vi "WPI_Camera HTTP Connection Respondervi.vi"(10 "parameters":T1(array[cluster]), 11 "connection ID":refnum<k5>) -> ()   [LabVIEW 2017]
doc: "This VI is launched each time a new client camera connection is requested. The connection will remain open until closed by the client or because of errors with the camera. Parameters are name/lvalue pairs that have been parsed from a URL request. Supported parameters are name, fps, resolution, compression, exposure, brightness, whitebalance, sharpness, and colorlevel.\n\nThe first four parameters are filled with defaults if not provided, but the latter four are only set if provided."
uses:
  <vilib>/Rock Robotics/SystemInterfaces/NetworkCommunication/NetComm_UsageReport_ResourceType.ctl
  <vilib>/Rock Robotics/WPI/Camera/WPI_CameraImageSize.ctl
  <vilib>/Utility/error.llb/Error Cluster From Error Code.vi
  <vilib>/ErrorRing/Error Ring.xnode
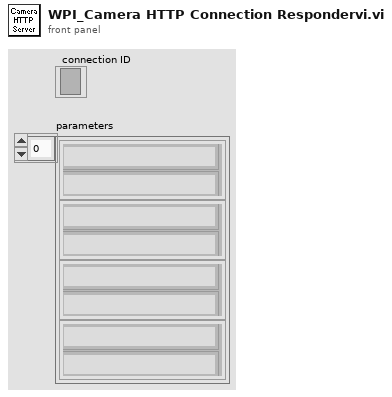
[diagram p1: front panel]
types:
  T1 = cluster{"token string":string, "token string 2":string}[]
  T2 = typedef "Image Type" = u32
  T3 = cluster{"White Balance":string, "Brightness":i32, "Sharpness":i32, "Saturation":i32, "Exposure":string}
  T4 = cluster{"Camera Name":string, "Size":string, "Frame Rate":i32, "Compression":i32}
  T5 = typedef "NetComm_UsageReport_ResourceType.ctl" = enum8{"Controller", "Module", "Language", "CANPlugin", "Accelerometer", "ADXL345", "AnalogChannel", "AnalogTrigger", "AnalogTriggerOutput", "CANJaguar", "Compressor", "Counter", "Dashboard", "DigitalInput", "DigitalOutput", "DriverStationCIO", "DriverStationEIO", "DriverStationLCD", "Encoder", "GearTooth", "Gyro", "I2C", "Framework", "Jaguar", "Joystick", "Kinect", "KinectStick", "PIDController", "Preferences", "PWM", "Relay", "RobotDrive", "SerialPort", "Servo", "Solenoid", "SPI", "Task", "Ultrasonic", "Victor", "Button", "Command", "AxisCamera", "PCVideoServer", "SmartDashboard", "Talon", "HiTechnicColorSensor", "HiTechnicAccel", "HiTechnicCompass", "SRF08", "AnalogOutput", "Victor SP", "Talon SRX", "CAN Talon SRX", "ADXL362 Accel", "ADXRS450 Gyro", "Rev SPARK", "Mindsensors SD540", "Digital Filter", "ADIS16448", "PDP", "PCM", "PigeonIMU", "Nidec Brushless", "CTRE CANifier", "CTRE Future 0", "CTRE Future 1", "CTRE Future 2", "CTRE Future 3", "CTRE Future 4", "CTRE Future 5", "CTRE Future 6"}
  T6 = cluster{"White Balance":bool, "Brightness":bool, "Sharpness":bool, "Saturation":bool, "Exposure":bool}
  T7 = typedef "WPI_CameraDevRef.ctl" = cluster{"Camera Address":string, "CameraStatus":errorcluster}
  T8 = typedef "IMAQ Image.ctl" = refnum<image>
  T9 = typedef "WPI_CameraImageSize.ctl" = enum16{"640x480", "320x240", "160x120", "Custom"}
  T10 = enum16{"Update Mode", "Get Image", "Get Image Data"}
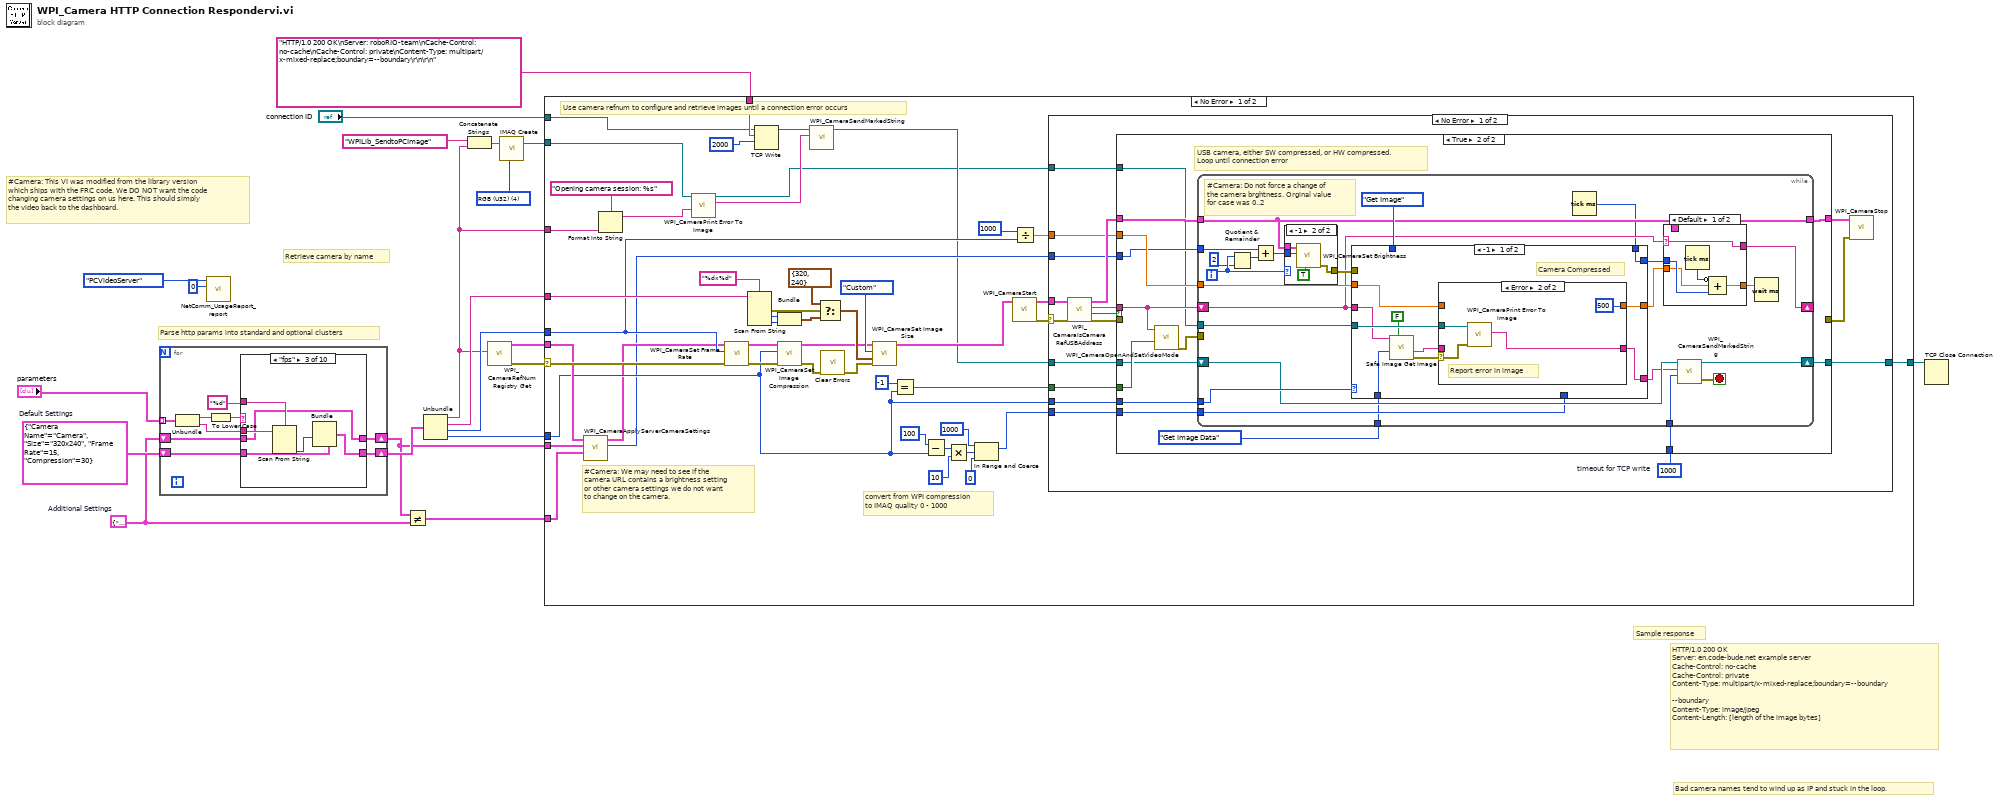
[diagram p0: block diagram]
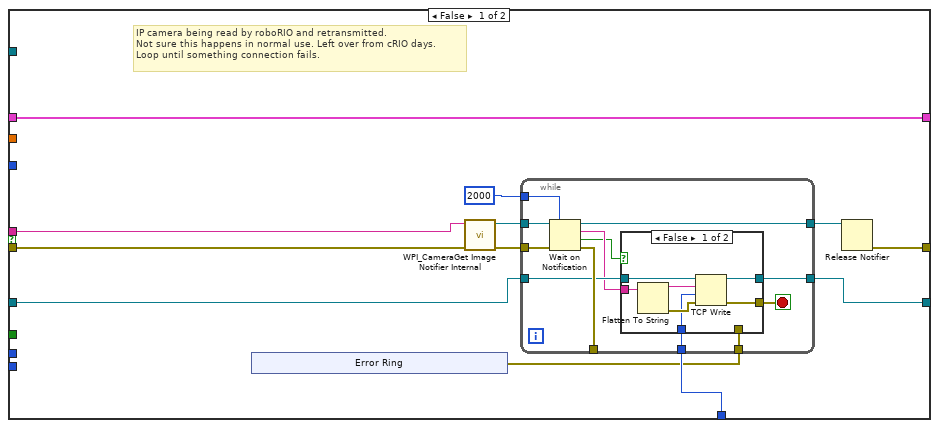
[diagram p2: hidden frame]
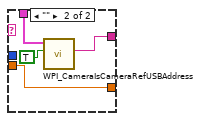
[diagram p4: hidden frame]
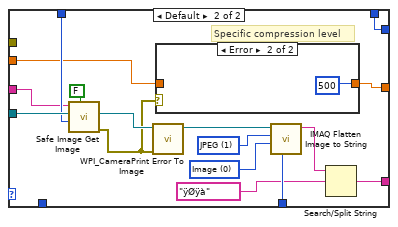
[diagram p7: hidden frame]
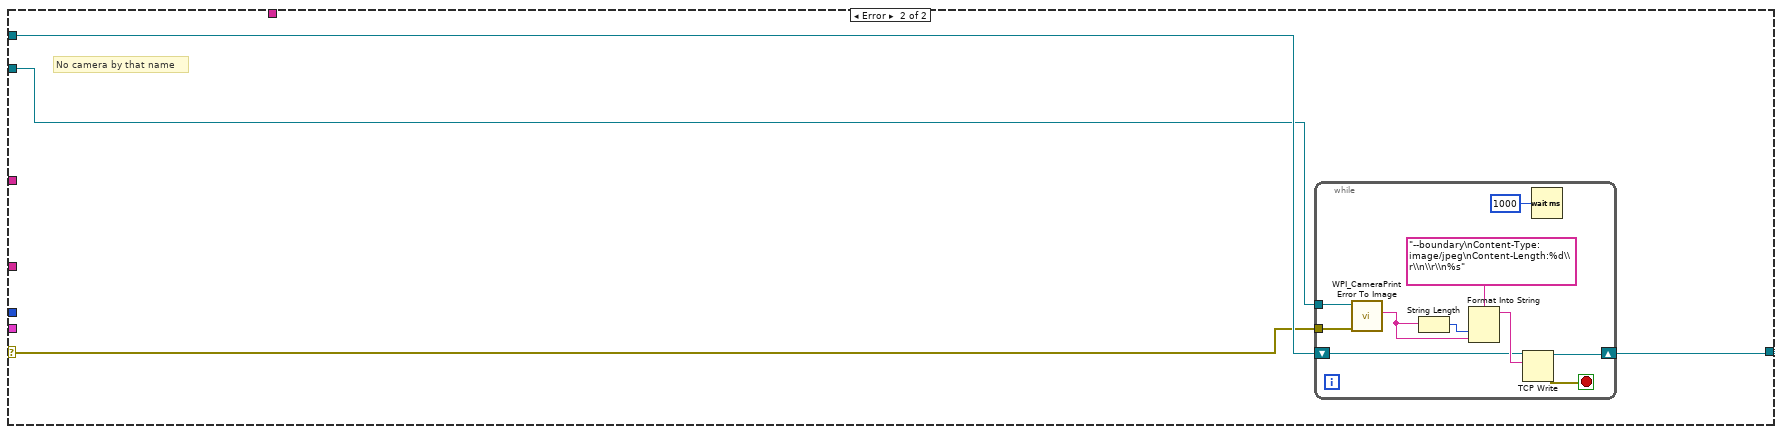
[diagram p10: hidden frame]
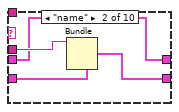
[diagram p12: hidden frame]
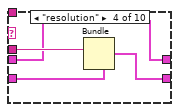
[diagram p13: hidden frame]
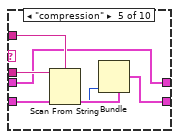
[diagram p14: hidden frame]
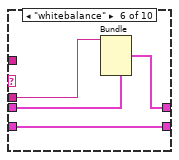
[diagram p15: hidden frame]
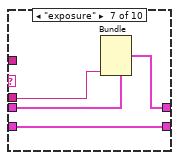
[diagram p16: hidden frame]
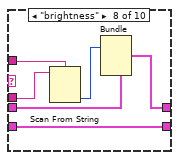
[diagram p17: hidden frame]
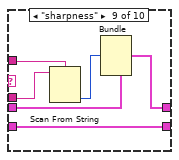
[diagram p18: hidden frame]
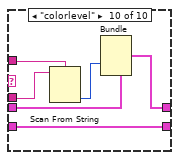
[diagram p19: hidden frame]
diagram:
  w4 = T2 4 items=["Grayscale (U8)", "Grayscale (I16)", "Grayscale (SGL)", "Complex (CSG)", "RGB (U32)", "HSL (U32)", "RGB (U64)", "Grayscale (U16)"] ("Image Type")
  w12 = T3 {"White Balance"="", "Brightness"=-1, "Sharpness"=-1, "Saturation"=-1, "Exposure"=""}  # Additional Settings
  w18 = T4 {"Camera Name"="Camera", "Size"="320x240", "Frame Rate"=15, "Compression"=30}  # Default Settings
  # "#Camera: This VI was modified from the library version\nwhich ships with the FRC code. We DO NOT want the code\nchanging camera settings on us here. This should simply\nthe video back to the dashboard."
  # "Sample response"
  # "HTTP/1.0 200 OK\nServer: en.code-bude.net example server\nCache-Control: no-cache\nCache-Control: private\nContent-Type: multipart/x-mixed-replace;boundary=--boundary\n \n--boundary\nContent-Type: image/jpeg\nContent-Length: [length of the image bytes]"
  # "Retrieve camera by name"
  # "Parse http params into standard and optional clusters"
  # "Bad camera names tend to wind up as IP and stuck in the loop."
  n1 = for {
    tunnel: "parameters" -> [w30] mode=indexing
    shift-right: [w25] -> w15
    shift-left: w18 -> [w27]
    shift-right: [w22] -> w10
    shift-left: w12 -> [w23]
    n2 = Unbundle(w30) -> ("token string"=w29:string, "token string 2"=w26:string)
    n3 = To Lower Case(string=w29) -> (all lower case string=w28:string)
    n4 = case shown="\"fps\"" w28 {
      tunnel: w27 -> [w32 w36 w42 w46 w52 w56 w60 w66 w72 w78]
      tunnel: w26 -> [_ w35 w40 w44 w50 w54 w57 w62 w68 w74]
      tunnel: [w32 w34 w41 w45 w51 w56 w60 w66 w72 w78] -> w25
      tunnel: "%d" -> [_ _ w39 _ w48 _ _ w63 w69 w75]
      tunnel: w23 -> [w31 w33 w37 w43 w47 w55 w59 w65 w71 w77]
      tunnel: [w31 w33 w37 w43 w47 w53 w58 w64 w70 w76] -> w22
      frame Default {
      }
      frame "name" {
        n5 = Bundle(cluster=w36, "Camera Name"=w35) -> (w34:T4)  [unwired: 3 in]
      }
      frame "fps" {
        n6 = Scan From String(format string=w39, input string=w40) -> (output 1=w38:i32)  [unwired: 3 in, 3 out]
        n7 = Bundle(cluster=w42, "Frame Rate"=w38) -> (w41:T4)  [unwired: 3 in]
      }
      frame "resolution" {
        n8 = Bundle(cluster=w46, "Size"=w44) -> (w45:T4)  [unwired: 3 in]
      }
      frame "compression" {
        n9 = Scan From String(format string=w48, input string=w50) -> (output 1=w49:i32)  [unwired: 3 in, 3 out]
        n10 = Bundle(cluster=w52, "Compression"=w49) -> (w51:T4)  [unwired: 3 in]
      }
      frame "whitebalance" {
        n11 = Bundle(cluster=w55, "White Balance"=w54) -> (w53:T3)  [unwired: 4 in]
      }
      frame "exposure" {
        n12 = Bundle(cluster=w59, "Exposure"=w57) -> (w58:T3)  [unwired: 4 in]
      }
      frame "brightness" {
        n13 = Scan From String(format string=w63, input string=w62) -> (output 1=w61:i32)  [unwired: 3 in, 3 out]
        n14 = Bundle(cluster=w65, "Brightness"=w61) -> (w64:T3)  [unwired: 4 in]
      }
      frame "sharpness" {
        n15 = Scan From String(format string=w69, input string=w68) -> (output 1=w67:i32)  [unwired: 3 in, 3 out]
        n16 = Bundle(cluster=w71, "Sharpness"=w67) -> (w70:T3)  [unwired: 4 in]
      }
      frame "colorlevel" {
        n17 = Scan From String(format string=w75, input string=w74) -> (output 1=w73:i32)  [unwired: 3 in, 3 out]
        n18 = Bundle(cluster=w77, "Saturation"=w73) -> (w76:T3)  [unwired: 4 in]
      }
    }
  }
  n19 = call <vilib>:"NetComm_UsageReport_report.vi"("Instance Number"=u8 0, "Resource Type"=NetComm_UsageReport_ResourceType."PCVideoServer") -> ()  [unwired: 10 in]
  n20 = Not Equal?(x=w10, y=w12) -> (x != y?=w11:T6)
  n21 = Unbundle(w15) -> ("Camera Name"=w2:string, "Size"=w16:string, "Frame Rate"=w8:i32, "Compression"=w9:i32)
  n22 = Concatenate Strings("WPILib_SendtoPCImage", w2) -> (w3:string)
  n23 = call <vilib>:"WPI_CameraRefNum Registry Get.vi"("refnum name"=w2) -> ("error out"=w6:errorcluster, "CameraDevRef"=w17:T7)  [unwired: 9 in]
  n24 = call "IMAQ Create"("Image Name"=w3, "Image Type"=w4) -> ("New Image"=w5:T8)  [unwired: 3 in, 1 out]
  n25 = case shown="No Error" w6 {
    selector: w6 -> [w102 w268]
    tunnel: [w126 w269] -> w21
    tunnel: w17 -> [w94 _]
    tunnel: w16 -> [w113 _]
    tunnel: w11 -> [w104 _]
    tunnel: w10 -> [w103 _]
    tunnel: w9 -> [w93 _]
    tunnel: w8 -> [w101 _]
    tunnel: "connection ID" -> [w81 w270]
    tunnel: w5 -> [w86 w267]
    tunnel: w2 -> [w88 _]
    tunnel: "HTTP/1.0 200 OK\nServer: roboRIO-team\nCache-Control: no-cache\nCache-Control: private\nContent-Type: multipart/x-mixed-replace;boundary=--boundary\r\n\r\n" ("regular expression") -> [w82 _]
    frame No Error {
      # "#Camera: We may need to see if the\ncamera URL contains a brightness setting\nor other camera settings we do not want\nto change on the camera."
      # "Use camera refnum to configure and retrieve images until a connection error occurs"
      # "convert from WPI compression\nto IMAQ quality 0 - 1000"
      n26 = call <vilib>:"WPI_CameraApplyServerCameraSettings.vi"("Unique"=w104, "Additional Settings"=w103, "CameraDevRef"=w94) -> ("Brightness"=w91:i32, "CameraDevRef Out"=w92:T7)  [unwired: 7 in]
      n27 = Format Into String(format string="Opening camera session: %s", w88) -> (resulting string=w84:string)  [unwired: 2 in, 1 out]
      n28 = call <vilib>:"WPI_CameraPrint Error To Image.vi"("String"=w84, "Image"=w86) -> ("flattened error string"=w90:string, "Image out"=w85:T8)  [unwired: 8 in]
      n29 = call <vilib>:"WPI_CameraSet Frame Rate.vi"("error in (no error)"=w102, "Frame Rate (fps)"=w101, "CameraDevRef"=w92) -> ("error out"=w98:errorcluster, "CameraDevRef Out"=w100:T7)  [unwired: 7 in]
      n30 = Scan From String(format string="%dx%d", input string=w113) -> (error out=w108:errorcluster, output 1=w111:i32, output 2=w110:i32)  [unwired: 4 in, 2 out]
      n31 = TCP Write(connection ID=w81, data in=w82, 9:2000) -> (connection ID out=w80:refnum<k5>)  [unwired: 1 in, 2 out]
      n32 = Bundle(w111, w110) -> (w107:cluster{i32, i32})  [unwired: 1 in]
      n33 = call <vilib>:"WPI_CameraSet Image Compression.vi"("error in (no error)"=w98, "Compression"=w93, "CameraDevRef"=w100) -> ("error out"=w97:errorcluster, "CameraDevRef Out"=w99:T7)  [unwired: 7 in]
      n34 = call <vilib>:"WPI_CameraSendMarkedString.vi"("Data String"=w90, "TCP Network Connection in"=w80) -> ("TCP Network Connection out"=w89:refnum<k5>)  [unwired: 8 in, 1 out]
      n35 = Select(t=cluster{i32, i32} {320, 240} ("s? t:f"), s=w108, f=w107) -> (s? t:f=w106:cluster{i32, i32})
      n36 = call <vilib>:"Clear Errors.vi"("error in (no error)"=w97) -> ("error out"=w96:errorcluster)  [unwired: 5 in, 1 out]
      n37 = call <vilib>:"WPI_CameraSet Image Size.vi"("error in (no error)"=w96, "Size W,H (pix)"=w106, "Image Size"=WPI_CameraImageSize."Custom", "CameraDevRef"=w99) -> ("CameraDevRef Out"=w95:T7)  [unwired: 6 in, 1 out]
      n38 = Equal?(x=-1, y=w93) -> (x = y?=w114:bool)
      n39 = Subtract(x=100, y=w93) -> (x-y=w118:i32)
      n40 = Multiply(x=w118, y=10) -> (x*y=w120:i32)
      n41 = In Range and Coerce(upper limit=1000, x=w120, lower limit=0) -> (coerced(x)=w116:i32)  [unwired: 1 out]
      n42 = call <vilib>:"WPI_CameraStart.vi"("CameraDevRef"=w95) -> ("error out"=w79:errorcluster, "CameraDevRef"=w125:T7)  [unwired: 1 in, 8 out]
      n43 = Divide(x=u16 1000 ("port"), y=w101) -> (x/y=w123:dbl)
      n44 = case shown="No Error" w79 {
        selector: w79 -> [w127 _]
        tunnel: [w143 w266] -> w126
        tunnel: w125 -> [w138 _]
        tunnel: w123 -> [w136 _]
        tunnel: w116 -> [w135 _]
        tunnel: w114 -> [w134 _]
        tunnel: w93 -> [w131 _]
        tunnel: w91 -> [w130 _]
        tunnel: w89 -> [w129 w266]
        tunnel: w85 -> [w128 _]
        frame No Error {
          w132 = 1000  # timeout for TCP write
          n45 = call <vilib>:"WPI_CameraIsCameraRefUSBAddress.vi"("error in (no error)"=w127, "CameraDevRef"=w138) -> ("error out"=w133:errorcluster, "USB?"=w139:bool, "Camera Address Out"=w140:string, "CameraDevRef out"=w137:T7)  [unwired: 6 in]
          n46 = case shown="True" w139 {
            tunnel: w129 -> [w155 w181]
            tunnel: [w154 w194] -> w143
            tunnel: w133 -> [w153 _]
            tunnel: w140 -> [w151 w190]
            tunnel: [w145 w192] -> w142
            tunnel: w137 -> [w145 w193]
            tunnel: [w149 _] -> w141
            tunnel: w135 -> [_ w187]
            tunnel: w136 -> [_ w185]
            tunnel: w131 -> [_ w191]
            tunnel: w134 -> [_ w189]
            tunnel: w132 -> [w147 w188]
            tunnel: w130 -> [_ w183]
            tunnel: w128 -> [_ w182]
            frame False {
              # "IP camera being read by roboRIO and retransmitted.\nNot sure this happens in normal use. Left over from cRIO days.\nLoop until something connection fails."
              n47 = xnode "Error Ring"() -> ("error out"=w144:errorcluster)
              n48 = call <vilib>:"WPI_CameraGet Image Notifier Internal.vi"("error in (no error)"=w153, "Camera Address"=w151) -> ("error out"=w152:errorcluster, "Image Notifier"=w150:refnum<notifier>)  [unwired: 8 out]
              n49 = while {
                tunnel: w152 -> [w171]
                tunnel: w155 -> [w166]
                tunnel: [w169] -> _
                tunnel: [w165] -> w154
                tunnel: w150 -> [w170]
                tunnel: [w168] -> w148
                tunnel: w147 -> [w167]
                tunnel: w144 -> [w162]
                tunnel: 2000 ("Timeout in ms (-1)") -> [w161]
                stop <- w160 stop-if-true
                n50 = Wait on Notification(notifier=w170, timeout in ms (-1)=w161, error in (no error)=w171) -> (notifier out=w168:refnum<notifier>, notification=w164:string, timed out?=w163:bool, error out=w169:errorcluster)  [unwired: 1 out]
                n51 = case shown="False" w163 {
                  tunnel: [w176 w179] -> w160
                  tunnel: w167 -> [w175 _]
                  tunnel: w166 -> [w174 w180]
                  tunnel: [w172 w180] -> w165
                  tunnel: w164 -> [w173 _]
                  tunnel: w162 -> [_ w179]
                  frame False {
                    n52 = Flatten To String(anything=w173) -> (data string=w178:string, error out=w177:errorcluster)  [unwired: 1 in, 3 out]
                    n53 = TCP Write(connection ID=w174, data in=w178, error in (no error)=w177, 9:w175) -> (connection ID out=w172:refnum<k5>, error out=w176:errorcluster)  [unwired: 1 out]
                  }
                  frame True {
                  }
                }
              }
              n54 = Release Notifier(notifier=w148) -> (error out=w149:errorcluster)  [unwired: 1 in, 3 out]
            }
            frame True {
              # "USB camera, either SW compressed, or HW compressed.\nLoop until connection error"
              n55 = call <vilib>:"WPI_CameraOpenAndSetVideoMode.vi"("USB JPEG"=w189, "Camera Address"=w190) -> ("error out"=w186:errorcluster)  [unwired: 9 in]
              n56 = while {
                shift-right: [w211] -> w194
                shift-left: w181 -> [w216]
                tunnel: [w201] -> w192
                tunnel: w193 -> [w201]
                tunnel: w191 -> [w218]
                tunnel: w188 -> [w215]
                tunnel: w187 -> [w214]
                tunnel: w186 -> [_]
                tunnel: w185 -> [w210]
                tunnel: T10."Get Image Data" ("Operation") -> [w209]
                tunnel: w183 -> [w207]
                shift-right: [w202] -> _
                shift-left: w190 -> [w200]
                tunnel: w182 -> [w199]
                i -> [w205]
                stop <- w212 stop-if-true
                # "#Camera: Do not force a change of\nthe camera brghtness. Orginal value\nfor case was 0..2"
                n57 = Quotient & Remainder(x=w205, y=u16 2 ("port")) -> (x-y*floor(x/y)=w206:i32)  [unwired: 1 out]
                n58 = Add(x=w207, y=w206) -> (x+y=w204:i32)
                n59 = case shown="-1" w205 {
                  tunnel: w201 -> [_ w231]
                  tunnel: [_ w230] -> w208
                  tunnel: w204 -> [_ w229]
                  frame Default {
                  }
                  frame -1 {
                    n60 = call <vilib>:"WPI_CameraSet Brightness.vi"("Force"=TRUE, "Brightness"=w229, "CameraDevRef"=w231) -> ("error out"=w230:errorcluster)  [unwired: 7 in, 1 out]
                  }
                }
                n61 = Tick Count (ms)() -> (millisecond timer value=w196:u32)
                n62 = case shown="-1" w218 {
                  tunnel: [w239 w258] -> w213
                  tunnel: w200 -> [w233 w250]
                  tunnel: w199 -> [w238 w260]
                  tunnel: w214 -> [_ w261]
                  tunnel: T10."Get Image" ("Operation") -> [_ w259]
                  tunnel: w210 -> [w237 w252]
                  tunnel: [w236 w251] -> w198
                  tunnel: w209 -> [w235 _]
                  tunnel: w208 -> [_ _]
                  tunnel: [w232 w249] -> w197
                  tunnel: w196 -> [w232 w249]
                  frame -1 {
                    # "Camera Compressed"
                    n63 = call <vilib>:"Safe Image Get Image.vi"("Wait"=FALSE ("DB"), "Operation"=w235, "Session In"=w233) -> ("error out"=w241:errorcluster, "Image Data String"=w240:string)  [unwired: 5 in, 2 out]
                    n64 = case shown="Error" w241 {
                      selector: w241 -> [_ w247]
                      tunnel: [w243 w244] -> w239
                      tunnel: w240 -> [w243 _]
                      tunnel: w238 -> [_ w246]
                      tunnel: w237 -> [w242 _]
                      tunnel: [w242 u16 500 ("port")] -> w236
                      frame No Error {
                      }
                      frame Error {
                        # "Report error in image"
                        n65 = call <vilib>:"WPI_CameraPrint Error To Image.vi"("error in (no error)"=w247, "Image"=w246) -> ("flattened error string"=w244:string)  [unwired: 8 in, 1 out]
                      }
                    }
                  }
                  frame Default {
                    w262 = 0 items=["Image", "Image and Vision Info", "Reference to Image"] ("Type of Flatten (Image and Vision Info)")
                    w263 = 1 items=["None", "JPEG", "PACKED BINARY"] ("Compression (None)")
                    # "Specific compression level"
                    n66 = call <vilib>:"Safe Image Get Image.vi"("Wait"=FALSE ("DB"), "Operation"=w259, "Image In"=w260, "Session In"=w250) -> ("error out"=w253:errorcluster, "Image Out"=w254:T8)  [unwired: 4 in, 2 out]
                    n67 = call <vilib>:"WPI_CameraPrint Error To Image.vi"("error in (no error)"=w253, "Image"=w254) -> ("Image out"=w256:T8)  [unwired: 8 in, 1 out]
                    n68 = case shown="Error" w253 {
                      tunnel: w252 -> [w264 _]
                      tunnel: [w264 500] -> w251
                      frame No Error {
                      }
                      frame Error {
                      }
                    }
                    n69 = call "IMAQ Flatten Image to String"("Quality (750)"=w261, "Type of Flatten (Image and Vision Info)"=w262, "Compression (None)"=w263, "Image"=w256) -> ("Data String"=w257:string)  [unwired: 6 in, 1 out]
                    n70 = Search/Split String(string=w257, search string/char (-)="ÿØÿà" ("format string")) -> (match + rest of string=w258:string)  [unwired: 1 in, 2 out]
                  }
                }
                n71 = case shown="Default" w200 {
                  selector: w200 -> [w223 _]
                  tunnel: w201 -> [_ w227]
                  tunnel: [w223 w226] -> w202
                  tunnel: w198 -> [w220 w224]
                  tunnel: w197 -> [w222 _]
                  tunnel: [w221 w224] -> w195
                  frame Default {
                    n72 = Tick Count (ms)() -> (millisecond timer value=w219:u32)
                    n73 = Compound Arithmetic op=ADD(invert w219, w220, w222) -> (w221:dbl)
                  }
                  frame "" {
                    n74 = call <vilib>:"WPI_CameraIsCameraRefUSBAddress.vi"("Enumerate"=TRUE ("Enumerate?"), "CameraDevRef"=w227) -> ("Camera Address Out"=w226:string)  [unwired: 6 in, 3 out]
                  }
                }
                n75 = call <vilib>:"WPI_CameraSendMarkedString.vi"("timeout for TCP write"=w215, "Data String"=w213, "TCP Network Connection in"=w216) -> ("error out"=w212:errorcluster, "TCP Network Connection out"=w211:refnum<k5>)  [unwired: 7 in]
                n76 = Wait (ms)(milliseconds to wait=w195) -> ()  [unwired: 1 out]
              }
            }
          }
          n77 = call <vilib>:"WPI_CameraStop.vi"("error in (no error)"=w141, "CameraDevRef"=w142) -> ()  [unwired: 10 out]
        }
        frame Error {
        }
      }
    }
    frame Error {
      # "No camera by that name"
      n78 = while {
        shift-right: [w275] -> w269
        shift-left: w270 -> [w274]
        tunnel: w268 -> [w273]
        tunnel: w267 -> [w272]
        stop <- w280 stop-if-true
        n79 = call <vilib>:"WPI_CameraPrint Error To Image.vi"("error in (no error)"=w273, "Image"=w272) -> ("flattened error string"=w278:string)  [unwired: 8 in, 1 out]
        n80 = String Length(string=w278) -> (length=w279:i32)
        n81 = Format Into String(format string="--boundary\nContent-Type: image/jpeg\nContent-Length:%d\\r\\n\\r\\n%s" ("regular expression"), w279, w278) -> (resulting string=w276:string)  [unwired: 2 in, 1 out]
        n82 = TCP Write(connection ID=w274, data in=w276) -> (connection ID out=w275:refnum<k5>, error out=w280:errorcluster)  [unwired: 2 in, 1 out]
        n83 = Wait (ms)(milliseconds to wait=u32 1000) -> ()  [unwired: 1 out]
      }
    }
  }
  n84 = TCP Close Connection(connection ID=w21) -> ()  [unwired: 1 in, 3 out]
